vi "冒泡排序法.vi"() -> ()   [LabVIEW 2018]
panel:
  in  "停止":bool
  out "单次过程":dbl[](graph)
  out "单步过程":cluster{i32[], i32[]}[](graph)
  out "结果图":dbl[][](graph)
  out "temp 2":dbl
  out "单步过程":dbl[](graph)
  out "单次过程":cluster{i32[], i32[]}[](graph)
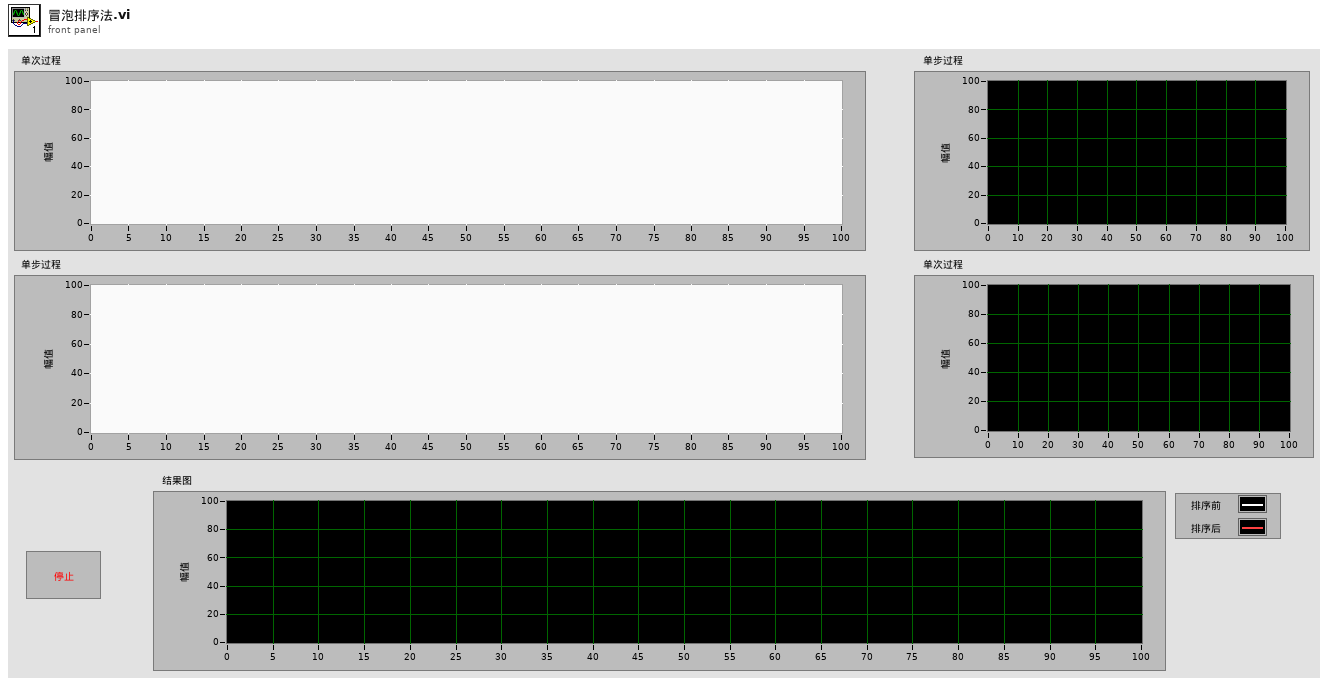
[diagram p1: front panel]
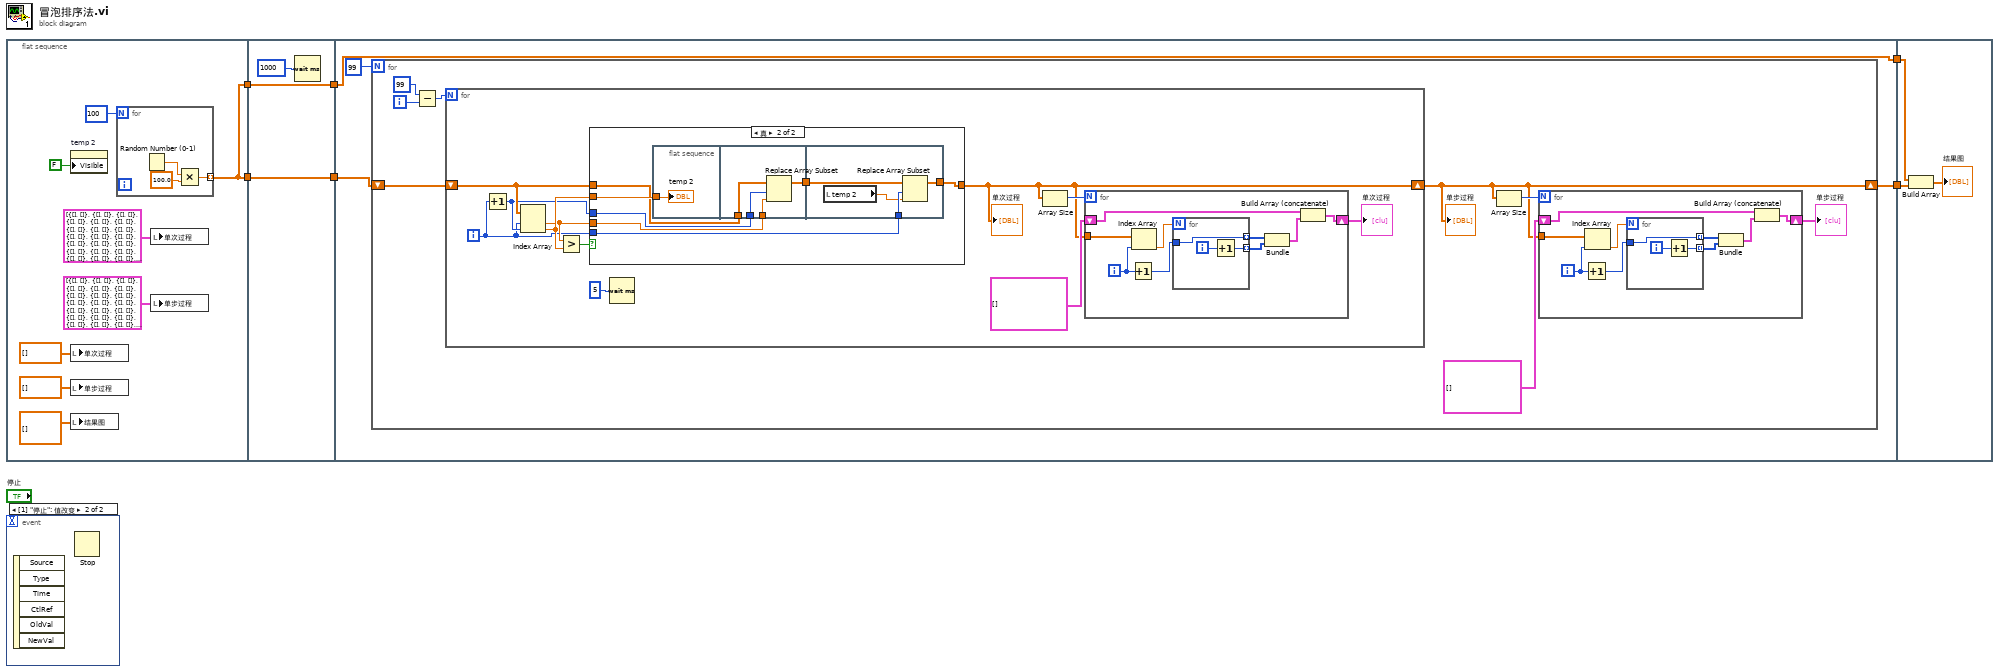
[diagram p0: block diagram]
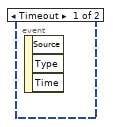
[diagram p2: hidden frame]
diagram:
  n1 = flat-sequence {
    tunnel: [w12] -> w4
    tunnel: [w12] -> w2
    tunnel: w4 -> [w20]
    tunnel: [w20] -> w3
    tunnel: w2 -> [w19]
    tunnel: [w19] -> w1
    tunnel: w3 -> [w21]
    tunnel: [w23] -> w6
    tunnel: w1 -> [w23]
    tunnel: [w22] -> w5
    tunnel: w6 -> [w86]
    tunnel: w5 -> [w85]
    frame #0 {
      n2 = property on="temp 2" class="DigNum (严格)"("Visible"=FALSE ("可见")) -> ()  [unwired: 2 in, 2 out]
      n3 = local write "单次过程"(dbl[] [] ("单次过程")) -> ()
      n4 = local write "单步过程"(dbl[] [] ("单步过程")) -> ()
      n5 = local write "结果图"(dbl[][] [] ("结果图")) -> ()
      n6 = for {
        N: 100 -> [_]
        tunnel: [w15] -> w12 mode=indexing
        n7 = Random Number (0-1)() -> (number: 0 to 1=w16:dbl)
        n8 = Multiply(x=w16, y=100.0) -> (x*y=w15:dbl)
      }
      n9 = local write "单次过程"(cluster{i32[], i32[]}[] [{[], []}, {[], []}, {[], []}, {[], []}, {[], []}, {[], []}, {[], []}, {[], []}, {[], []}, {[], []}, {[], []}, {[], []}, {[], []}, {[], []}, {[], []}, {[], []}, {[], []}, {[], []}, {[], []}, {[], []}, {[], []}, {[], []}, {[], []}, {[], []}, {[], []}, {[], []}, {[], []}, {[], []}, {[], []}, {[], []}, {[], []}, {[], []}, {[], []}, {[], []}, {[], []}, {[], []}, {[], []}, {[], []}, {[], []}, {[], []}, {[], []}, {[], []}, {[], []}, {[], []}, {[], []}, {[], []}, {[], []}, {[], []}, {[], []}, {[], []}, {[], []}, {[], []}, {[], []}, {[], []}, {[], []}, {[], []}, {[], []}, {[], []}, {[], []}, {[], []}, {[], []}, {[], []}, {[], []}, {[], []}, {[], []}, {[], []}, {[], []}, {[], []}, {[], []}, {[], []}, {[], []}, {[], []}, {[], []}, {[], []}, {[], []}, {[], []}, {[], []}, {[], []}, {[], []}, {[], []}, {[], []}, {[], []}, {[], []}, {[], []}, {[], []}, {[], []}, {[], []}, {[], []}, {[], []}, {[], []}, {[], []}, {[], []}, {[], []}, {[], []}, {[], []}, {[], []}, {[], []}, {[], []}, {[], []}, {[], []}] ("单次过程")) -> ()
      n10 = local write "单步过程"(cluster{i32[], i32[]}[] [{[], []}, {[], []}, {[], []}, {[], []}, {[], []}, {[], []}, {[], []}, {[], []}, {[], []}, {[], []}, {[], []}, {[], []}, {[], []}, {[], []}, {[], []}, {[], []}, {[], []}, {[], []}, {[], []}, {[], []}, {[], []}, {[], []}, {[], []}, {[], []}, {[], []}, {[], []}, {[], []}, {[], []}, {[], []}, {[], []}, {[], []}, {[], []}, {[], []}, {[], []}, {[], []}, {[], []}, {[], []}, {[], []}, {[], []}, {[], []}, {[], []}, {[], []}, {[], []}, {[], []}, {[], []}, {[], []}, {[], []}, {[], []}, {[], []}, {[], []}, {[], []}, {[], []}, {[], []}, {[], []}, {[], []}, {[], []}, {[], []}, {[], []}, {[], []}, {[], []}, {[], []}, {[], []}, {[], []}, {[], []}, {[], []}, {[], []}, {[], []}, {[], []}, {[], []}, {[], []}, {[], []}, {[], []}, {[], []}, {[], []}, {[], []}, {[], []}, {[], []}, {[], []}, {[], []}, {[], []}, {[], []}, {[], []}, {[], []}, {[], []}, {[], []}, {[], []}, {[], []}, {[], []}, {[], []}, {[], []}, {[], []}, {[], []}, {[], []}, {[], []}, {[], []}, {[], []}, {[], []}, {[], []}, {[], []}, {[], []}] ("单步过程")) -> ()
    }
    frame #1 {
      n11 = Wait (ms)(milliseconds to wait=u32 1000 ("等待时间（毫秒）")) -> ()  [unwired: 1 out]
    }
    frame #2 {
      n12 = for {
        N: 99 -> [_]
        shift-right: [w25] -> w22
        shift-left: w21 -> [w29]
        i -> [w32]
        n13 = Subtract(x=99, y=w32) -> (x-y=w30:i32)
        n14 = for {
          N: w30 -> [_]
          shift-right: [w45] -> w25
          shift-left: w29 -> [w52]
          i -> [w50]
          n15 = Increment(x=w50) -> (x+1=w51:i32)
          n16 = Index Array(array=w52, index #1=w50, index #2=w51) -> (element #1=w54:dbl, element #2=w55:dbl)
          n17 = Greater?(x=w54, y=w55) -> (0:w53:bool)
          n18 = case shown="真" w53 {
            tunnel: w55 -> [_ w75]
            tunnel: w52 -> [w68 w74]
            tunnel: w51 -> [_ w73]
            tunnel: w54 -> [_ w72]
            tunnel: w50 -> [_ w70]
            tunnel: [w68 w69] -> w45
            frame False {
            }
            frame True {
              n19 = flat-sequence {
                tunnel: w75 -> [w76]
                tunnel: w74 -> [w78]
                tunnel: w73 -> [w80]
                tunnel: w72 -> [w79]
                tunnel: [w77] -> w71
                tunnel: w71 -> [w84]
                tunnel: w70 -> [w83]
                tunnel: [w81] -> w69
                frame #0 {
                  "temp 2" <- w76
                }
                frame #1 {
                  n20 = Replace Array Subset(array=w78, new element=w79, index=w80) -> (w77:dbl[])
                }
                frame #2 {
                  n21 = local read "temp 2"() -> (w82:dbl)
                  n22 = Replace Array Subset(array=w84, new element=w82, index=w83) -> (w81:dbl[])
                }
              }
            }
          }
          "单次过程" <- w45
          n23 = Wait (ms)(milliseconds to wait=u32 5 ("等待时间（毫秒）")) -> ()  [unwired: 1 out]
          n24 = Array Size(array=w45) -> (size(s)=w47:i32)
          n25 = for {
            N: w47 -> [_]
            tunnel: w45 -> [w58]
            shift-right: [w60] -> w48
            shift-left: cluster{i32[], i32[]}[] [] -> [w59]
            i -> [w57]
            n26 = Increment(x=w57) -> (x+1=w63:i32)
            n27 = Index Array(array=w58, index=w57) -> (element=w56:dbl)
            n28 = for {
              N: w56 -> [_]
              tunnel: [w67] -> w64 mode=indexing
              tunnel: w63 -> [w67]
              tunnel: [w65] -> w62 mode=indexing
              i -> [w66]
              n29 = Increment(x=w66) -> (x+1=w65:i32)
            }
            n30 = Bundle(w64, w62) -> (w61:cluster{i32[], i32[]})  [unwired: 1 in]
            n31 = Build Array (concatenate)(w59, w61) -> (w60:cluster{i32[], i32[]}[])
          }
          "单次过程" <- w48
        }
        "单步过程" <- w25
        n32 = Array Size(array=w25) -> (size(s)=w27:i32)
        n33 = for {
          N: w27 -> [_]
          tunnel: w25 -> [w35]
          shift-right: [w37] -> w28
          shift-left: cluster{i32[], i32[]}[] [] -> [w36]
          i -> [w34]
          n34 = Increment(x=w34) -> (x+1=w40:i32)
          n35 = Index Array(array=w35, index=w34) -> (element=w33:dbl)
          n36 = for {
            N: w33 -> [_]
            tunnel: [w44] -> w41 mode=indexing
            tunnel: w40 -> [w44]
            tunnel: [w42] -> w39 mode=indexing
            i -> [w43]
            n37 = Increment(x=w43) -> (x+1=w42:i32)
          }
          n38 = Bundle(w41, w39) -> (w38:cluster{i32[], i32[]})  [unwired: 1 in]
          n39 = Build Array (concatenate)(w36, w38) -> (w37:cluster{i32[], i32[]}[])
        }
        "单步过程" <- w28
      }
    }
    frame #3 {
      n40 = Build Array(w86, w85) -> (→"结果图":dbl[][])
    }
  }
  n41 = event shown="[1] \"停止\": 值改变" {
    selector: _ -> [_ _]
    dyn-events: _ -> [_ _]
    timeout: _ -> [_ _]
    event Timeout {
      n42 = event-data() -> ()  [unwired: 1 in, 3 out]
    }
    event "停止": Value Change {
      n43 = event-data() -> ()  [unwired: 1 in, 6 out]
      n44 = Stop() -> ()  [unwired: 1 in]
    }
  }
